vi "CAvatappi Efficiency.vi"() -> ()   [LabVIEW 2017]
uses:
  <vilib>/Waveform/WDTFileIO.llb/Export Waveforms To Spreadsheet File (1D).vi
panel:
  in  "Displacement Scale (mm/V)":dbl
  out "Disp":dynamicdata(graph)
  out "Measured pressure":dynamicdata(graph)
  in  "stop":bool
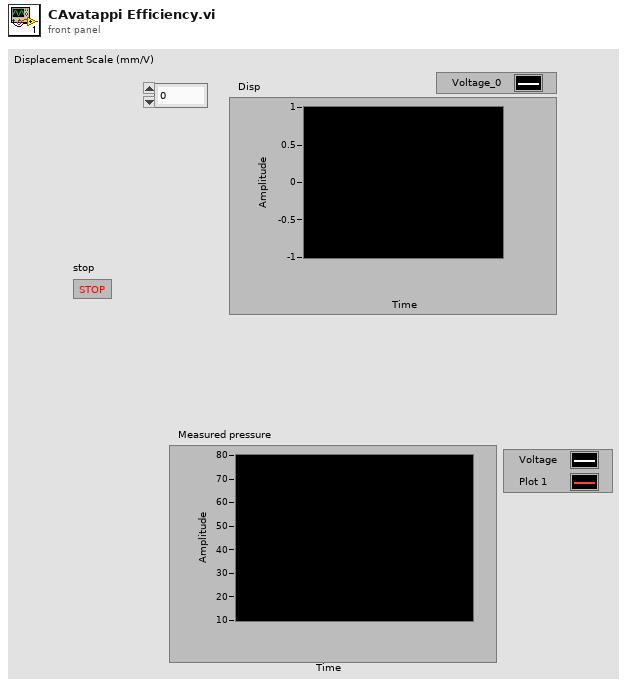
[diagram p1: front panel]
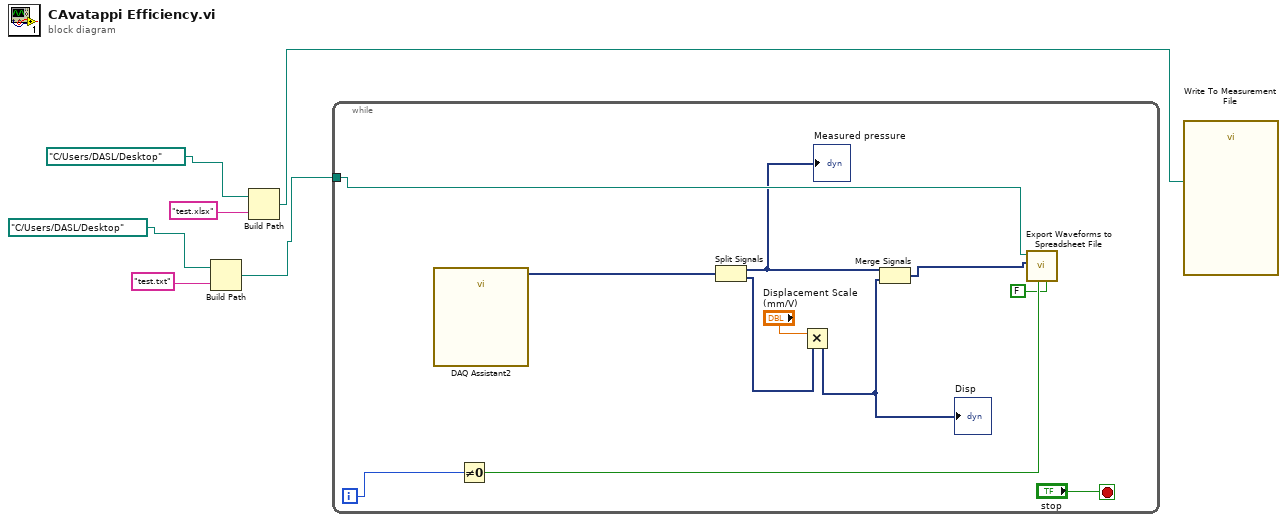
[diagram p0: block diagram]
diagram:
  n1 = Build Path(base path=path "C:/Users/DASL/Desktop", name or relative path="test.txt") -> (appended path=w1:path)
  n2 = Build Path(base path=path "C:/Users/DASL/Desktop", name or relative path="test.xlsx") -> (appended path=w4:path)
  n3 = while {
    tunnel: w1 -> [w12]
    i -> [w13]
    stop <- "stop" stop-if-true
    n4 = call "DAQ Assistant2"() -> ("data"=w7:dynamicdata)  [unwired: 17 in, 2 out]
    n5 = Not Equal To 0?(x=w13) -> (x != 0?=w10:bool)
    n6 = Split Signals(w7) -> (w8:dynamicdata, w14:dynamicdata)  [unwired: 2 in]
    "Measured pressure" <- w8
    n7 = Multiply(x="Displacement Scale (mm/V)", y=w14) -> (x*y=w15:dynamicdata)
    "Disp" <- w15
    n8 = Merge Signals(w8, w15) -> (w11:dynamicdata)
    n9 = call-poly <vilib>:"Export Waveforms to Spreadsheet File.vi"("header? (write header:T)"=FALSE, "append to file? (new file:F)"=w10, "waveforms"=w11, "file path (dialog if empty)"=w12) -> ()  [unwired: 6 in, 2 out]
  }
  n10 = call "Write To Measurement File"("Filename"=w4) -> ()  [unwired: 16 in, 3 out]
